vi "robot.vi"(1 "Robot Radius":dbl(slide)=1.0204081632653061 scale=0.0..10.0, 2 "direction":dbl(slide) scale=3.2..-3.2) -> (0 "output cluster":cluster{dbl[], dbl[]})   [LabVIEW 2009]
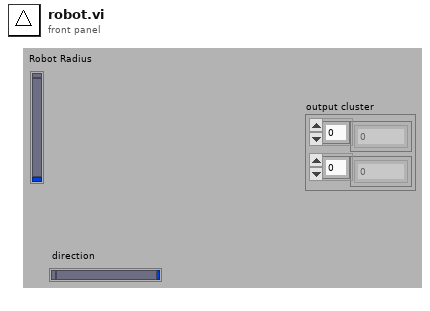
[diagram p1: front panel]
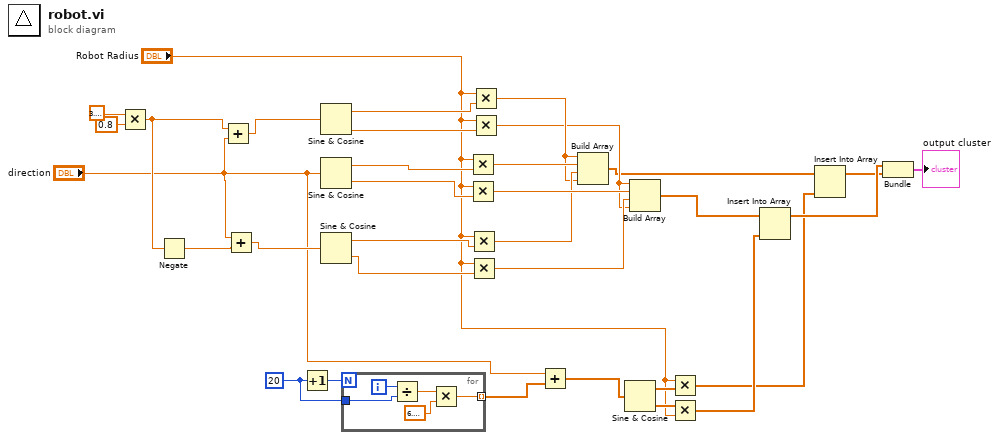
[diagram p0: block diagram]
diagram:
  w13 = 20
  n1 = Multiply(x=3.141592653589793, y=0.8) -> (x*y=w16:dbl)
  n2 = Negate(x=w16) -> (-x=w18:dbl)
  n3 = Add(x=w16, y="direction") -> (x+y=w15:dbl)
  n4 = Add(x="direction", y=w18) -> (x+y=w17:dbl)
  n5 = Increment(x=w13) -> (x+1=w14:i32)
  n6 = Sine & Cosine(0:w15) -> (1:w28:dbl, 2:w27:dbl)
  n7 = Sine & Cosine(0:"direction") -> (1:w33:dbl, 2:w32:dbl)
  n8 = Sine & Cosine(0:w17) -> (1:w26:dbl, 2:w25:dbl)
  n9 = for {
    N: w14 -> [_]
    tunnel: w13 -> [w37]
    tunnel: [w34] -> w2 mode=indexing
    i -> [w38]
    n10 = Divide(x=w38, y=w37) -> (x/y=w36:dbl)
    n11 = Multiply(x=w36, y=6.283185307179586) -> (x*y=w34:dbl)
  }
  n12 = Multiply(x="Robot Radius", y=w33) -> (x*y=w24:dbl)
  n13 = Multiply(x="Robot Radius", y=w32) -> (x*y=w31:dbl)
  n14 = Multiply(x="Robot Radius", y=w26) -> (x*y=w22:dbl)
  n15 = Multiply(x="Robot Radius", y=w25) -> (x*y=w23:dbl)
  n16 = Multiply(x="Robot Radius", y=w28) -> (x*y=w20:dbl)
  n17 = Multiply(x="Robot Radius", y=w27) -> (x*y=w19:dbl)
  n18 = Add(x="direction", y=w2) -> (x+y=w1:dbl[])
  n19 = Build Array(w20, w24, w22, w20) -> (w6:dbl[])
  n20 = Sine & Cosine(0:w1) -> (1:w12:dbl[], 2:w11:dbl[])
  n21 = Build Array(w19, w31, w23, w19) -> (w8:dbl[])
  n22 = Multiply(x="Robot Radius", y=w12) -> (x*y=w5:dbl[])
  n23 = Multiply(x=w11, y="Robot Radius") -> (x*y=w9:dbl[])
  n24 = Insert Into Array(array=w8, new element=w9) -> (w7:dbl[])  [unwired: 1 in]
  n25 = Insert Into Array(array=w6, new element=w5) -> (w4:dbl[])  [unwired: 1 in]
  n26 = Bundle(w7, w4) -> (→"output cluster":cluster{dbl[], dbl[]})  [unwired: 1 in]
